vi "Post-Build Package Modifications.vi"(8 "error in (no error)":errorcluster, 11 "Package File Path":path) -> (0 "error out":errorcluster)   [LabVIEW 2015]
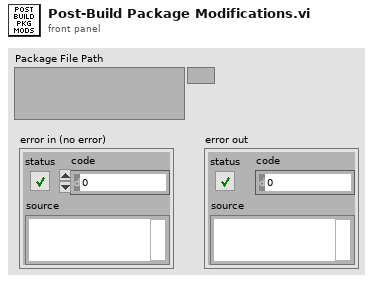
[diagram p1: front panel]
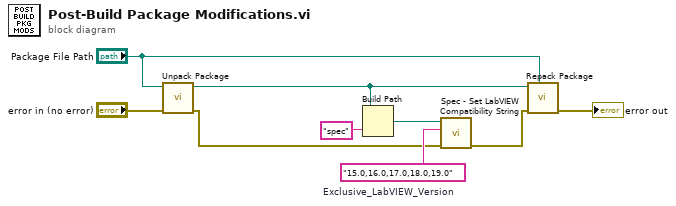
[diagram p0: block diagram]
diagram:
  w8 = "15.0,16.0,17.0,18.0,19.0"  # Exclusive_LabVIEW_Version
  n1 = call "Unpack Package.vi"("error in (no error)"="error in (no error)", "Package File"="Package File Path") -> ("error out"=w5:errorcluster, "Unpacked Package Directory"=w2:path)  [unwired: 7 in, 1 out]
  n2 = Build Path(base path=w2, name or relative path="spec" ("internal name (same as target)")) -> (appended path=w4:path)
  n3 = call "Spec - Set LabVIEW Compatibility String.vi"("error in (no error)"=w5, "Exclusive_LabVIEW_Version"=w8, "spec path"=w4) -> ("error out"=w6:errorcluster)  [unwired: 8 in]
  n4 = call "Repack Package.vi"("Package File (\"\": use name of directory to repack)"="Package File Path", "error in (no error)"=w6, "Directory to repack"=w2) -> ("error out"=→"error out":errorcluster)  [unwired: 8 in]
